vi "exist_svi.vi"(0 "Name":string, 2 "IN VARIANT":variant, 5 "error in (no error)":errorcluster, 12 "Create ?":bool) -> (14 "Name":string, 15 "index of element":i32, 16 "Exist":bool, 19 "error out":errorcluster)   [LabVIEW 2015]
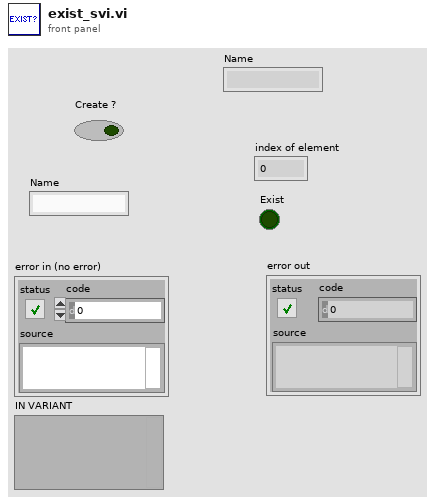
[diagram p1: front panel]
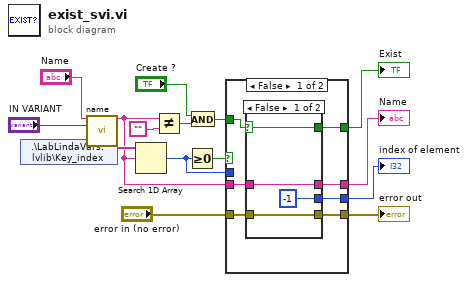
[diagram p0: block diagram]
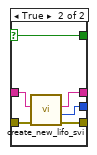
[diagram p2: hidden frame]
diagram:
  n1 = shared-variable ".\\LabLindaVars.lvlib\\Key_index"() -> (w15:string[])  [unwired: 1 in, 1 out]
  n2 = call "name.vi"("Name in"="Name", "IN VARIANT in"="IN VARIANT") -> ("Name"=w3:string)  [unwired: 12 in, 1 out]
  n3 = Search 1D Array(1D array=w15, element=w3) -> (index of element=w12:i32)  [unwired: 1 in]
  n4 = Not Equal?(x=w3, y="") -> (x != y?=w4:bool)
  n5 = Greater Or Equal To 0?(x=w12) -> (x >= 0?=w14:bool)
  n6 = And(x="Create ?", y=w4) -> (x .and. y?=w1:bool)
  n7 = case shown="False" w14 {
    selector: w14 -> [_ w34]
    tunnel: w3 -> [w22 w36]
    tunnel: [w16 w36] -> w10
    tunnel: w12 -> [_ w35]
    tunnel: [w17 w35] -> w13
    tunnel: w1 -> [w21 _]
    tunnel: [w20 w34] -> w11
    tunnel: "error in (no error)" -> [w19 w33]
    tunnel: [w18 w33] -> w8
    frame False {
      n8 = case shown="False" w21 {
        selector: w21 -> [w26 w31]
        tunnel: w22 -> [w23 w32]
        tunnel: [w26 w31] -> w20
        tunnel: w19 -> [w25 w30]
        tunnel: [w25 w29] -> w18
        tunnel: [-1 w28] -> w17
        tunnel: [w23 w27] -> w16
        frame False {
        }
        frame True {
          n9 = call "create_new_lifo_svi.vi"("error in (no error)"=w30, "Name in"=w32) -> ("error out"=w29:errorcluster, "Key Index"=w28:i32, "Name Out"=w27:string)  [unwired: 7 in]
        }
      }
    }
    frame True {
    }
  }
  "Exist" <- w11
  "index of element" <- w13
  "Name" <- w10
  "error out" <- w8
